vi "Convert Pinpad To String.vi"(10 "Pinpad":T1, 11 "Screen in":string) -> (1 "E":bool, 3 "Screen out":string)   [LabVIEW 2017]
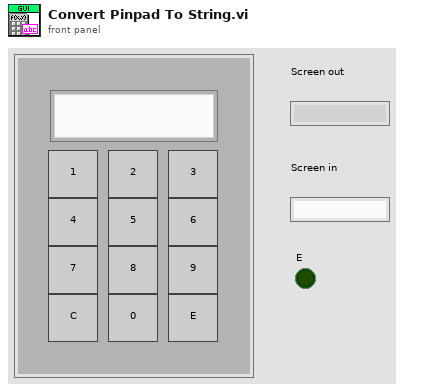
[diagram p1: front panel]
types:
  T1 = cluster{"Screen":string, "num1":bool, "num2":bool, "num3":bool, "num6":bool, "num5":bool, "num4":bool, "num7":bool, "num8":bool, "num9":bool, "C":bool, "num0":bool, "E":bool}
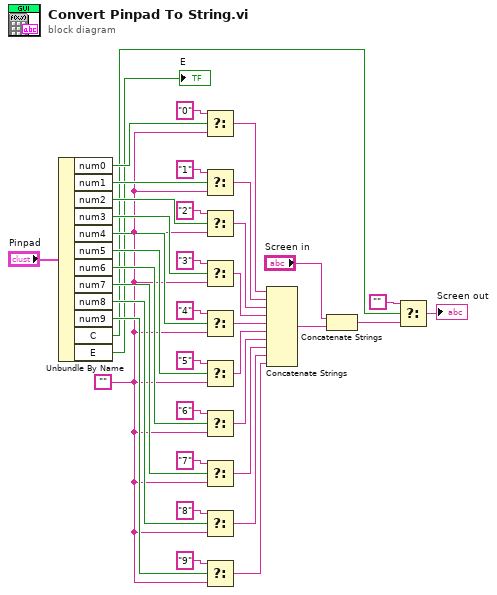
[diagram p0: block diagram]
diagram:
  w18 = ""
  n1 = Unbundle By Name("Pinpad") -> ("num0"=w38:bool, "num1"=w37:bool, "num2"=w36:bool, "num3"=w34:bool, "num4"=w33:bool, "num5"=w32:bool, "num6"=w35:bool, "num7"=w31:bool, "num8"=w30:bool, "num9"=w29:bool, "C"=w7:bool, "E"=→"E":bool)
  n2 = Select(t="0", s=w38, f=w18) -> (s? t:f=w17:string)
  n3 = Select(t="1", s=w37, f=w18) -> (s? t:f=w16:string)
  n4 = Select(t="2", s=w36, f=w18) -> (s? t:f=w15:string)
  n5 = Select(t="3", s=w34, f=w18) -> (s? t:f=w14:string)
  n6 = Select(t="4", s=w33, f=w18) -> (s? t:f=w13:string)
  n7 = Select(t="5", s=w32, f=w18) -> (s? t:f=w12:string)
  n8 = Select(t="6", s=w35, f=w18) -> (s? t:f=w11:string)
  n9 = Select(t="7", s=w31, f=w18) -> (s? t:f=w10:string)
  n10 = Select(t="8", s=w30, f=w18) -> (s? t:f=w9:string)
  n11 = Select(t="9", s=w29, f=w18) -> (s? t:f=w8:string)
  n12 = Concatenate Strings(w17, w16, w15, w14, w13, w12, w11, w10, w9, w8) -> (w3:string)
  n13 = Concatenate Strings("Screen in", w3) -> (w2:string)
  n14 = Select(t="", s=w7, f=w2) -> (s? t:f=→"Screen out":string)
